vi "com core.vi"(5 "VISA Resource":refnum<visa-resource-name>="COM4", 6 "Coil value":bool, 7 "功能":T1(ring), 8 "error in (no error)":errorcluster, 9 "HR values":u16[](array[numeric]), 10 "quantity":u16, 11 "starting address":u16) -> (0 "error out":errorcluster, 2 "Coils":bool[](array[boolean]), 3 "Registers":u16[](array[numeric]))   [LabVIEW 2016, in "一代CodMn.lvlib"]
uses:
  <vilib>/Plasmionique/MB Master/MB_Master_Serial/MB_Master_Serial.lvclass
  C:/Program Files (x86)/National Instruments/LabVIEW 2016/vi.lib/Plasmionique/MB Master/MB_Master/MB_Master.lvclass
  <vilib>/Plasmionique/MB Master/MB Master.lvlib
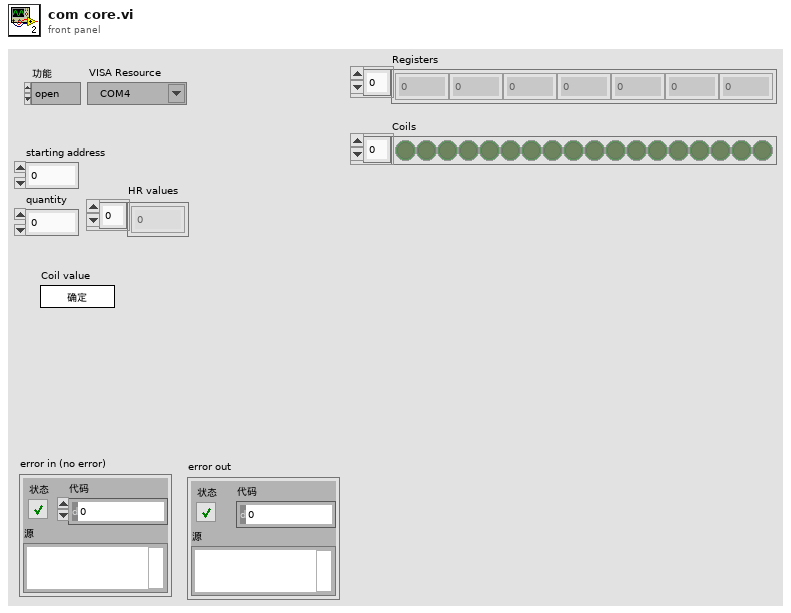
[diagram p1: front panel]
types:
  T1 = enum16{"open", "close", "readHR", "writeHR", "readCoil", "writeCoil"}
  T2 = cluster{"baud rate (bps)":u32, "stop bits":u16, "parity":u16, "flow control":u16, "timeout":u32, "retries":i32}
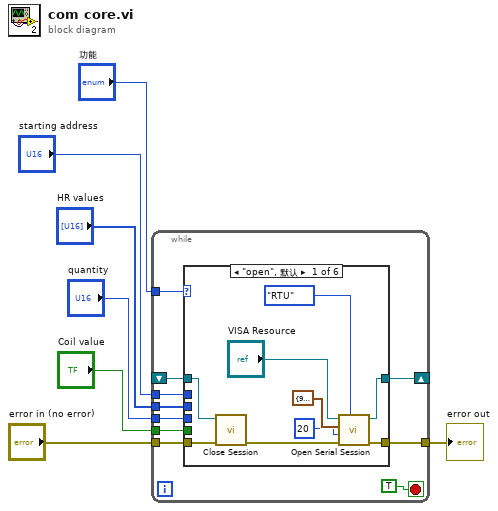
[diagram p0: block diagram]
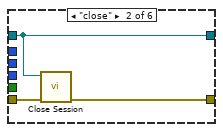
[diagram p2: hidden frame]
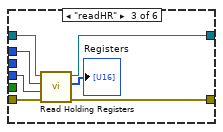
[diagram p3: hidden frame]
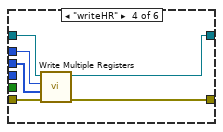
[diagram p4: hidden frame]
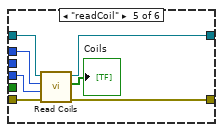
[diagram p5: hidden frame]
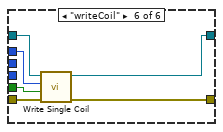
[diagram p6: hidden frame]
diagram:
  n1 = while {
    tunnel: "功能" -> [w16]
    shift-right: [w15] -> _
    shift-left: _ -> [w14]
    tunnel: [w13] -> w3
    tunnel: "error in (no error)" -> [w12]
    tunnel: "starting address" -> [w11]
    tunnel: "quantity" -> [w10]
    tunnel: "HR values" -> [w9]
    tunnel: "Coil value" -> [w8]
    stop <- TRUE stop-if-true
    n2 = case shown="\"open\", 默认" w16 {
      tunnel: [w25 w27 w35 w38 w45 w52] -> w15
      tunnel: w14 -> [w24 w27 w36 w42 w49 w54]
      tunnel: [w19 w28 w30 w37 w44 w51] -> w13
      tunnel: w12 -> [w18 w29 w34 w41 w48 w55]
      tunnel: w11 -> [_ _ w32 w40 w47 w53]
      tunnel: w10 -> [_ _ w31 _ w46 _]
      tunnel: w9 -> [_ _ _ w39 _ _]
      tunnel: w8 -> [_ _ _ _ _ w50]
      frame "open", Default {
        n3 = call-dynamic "Close Session.vi"("error in (no error)"=w18, "MB_Serial session"=w24) -> ("error out"=w23:errorcluster)  [unwired: 9 in]
        n4 = call <vilib>:"Open Serial Session.vi"("Mode (RTU)"=enum16{"RTU", "ASCII"}."RTU", "Error in"=w23, "Slave ID"=u8 20, "Serial Config"=T2 {"baud rate (bps)"=9600, "stop bits"=10, "parity"=0, "flow control"=0, "timeout"=500, "retries"=1}, "VISA Resource"="VISA Resource") -> ("Error out"=w19:errorcluster, "MB_Serial session"=w25:refnum<class "MB_Master_Serial.lvclass">)  [unwired: 5 in]
      }
      frame "close" {
        n5 = call-dynamic "Close Session.vi"("error in (no error)"=w29, "MB_Serial session"=w27) -> ("error out"=w28:errorcluster)  [unwired: 9 in]
      }
      frame "readHR" {
        n6 = call <vilib>:"Read Holding Registers.vi"("error in (no error)"=w34, "quantity"=w31, "starting address"=w32, "MB session in"=w36) -> ("error out"=w30:errorcluster, "Registers"=→"Registers":u16[], "MB session out"=w35:refnum<class "MB_Master_Serial.lvclass">)  [unwired: 5 in]
      }
      frame "writeHR" {
        n7 = call <vilib>:"Write Multiple Registers.vi"("error in (no error)"=w41, "values"=w39, "starting address"=w40, "MB session in"=w42) -> ("error out"=w37:errorcluster, "MB session out"=w38:refnum<class "MB_Master_Serial.lvclass">)  [unwired: 6 in]
      }
      frame "readCoil" {
        n8 = call <vilib>:"Read Coils.vi"("error in (no error)"=w48, "quantity"=w46, "starting address"=w47, "MB session in"=w49) -> ("error out"=w44:errorcluster, "Coils"=→"Coils":bool[], "MB session out"=w45:refnum<class "MB_Master_Serial.lvclass">)  [unwired: 5 in]
      }
      frame "writeCoil" {
        n9 = call <vilib>:"Write Single Coil.vi"("error in (no error)"=w55, "value"=w50, "address"=w53, "MB session in"=w54) -> ("error out"=w51:errorcluster, "MB session out"=w52:refnum<class "MB_Master_Serial.lvclass">)  [unwired: 6 in]
      }
    }
  }
  "error out" <- w3
